vi "Event Teardown.vi"(11 "Event Teardown in":refnum<class "Event Teardown.lvclass">) -> (3 "Event Teardown out":refnum<class "Event Teardown.lvclass">)   [LabVIEW 2021, in "Event Teardown.lvlib" / "Event Teardown.lvclass"]
uses:
  Event Teardown.lvclass
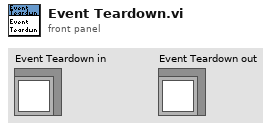
[diagram p1: front panel]
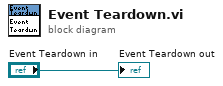
[diagram p0: block diagram]
diagram:
  "Event Teardown out" <- "Event Teardown in"
